vi "Claw Control.vi"() -> ()   [LabVIEW 2014]
doc: "This VI runs in parallel to other tasks. It can contain as many user-defined periodic loops as you need. These can carry out PID or other sorts of timed response."
uses:
  Vision/Robot Global Data.vi
  <vilib>/Rock Robotics/Network Tables/SD Write Number.vi
  <vilib>/Rock Robotics/Network Tables/SD Write Boolean.vi
panel:
  in  "PDB Channel":dbl
  out "Claw Motor Current Chart":dbl(graph)
  out "Time Request Running":u32
  out "Start Time":u32
  out "Prior Claw State":dbl
  out "Claw State":dbl=2.0
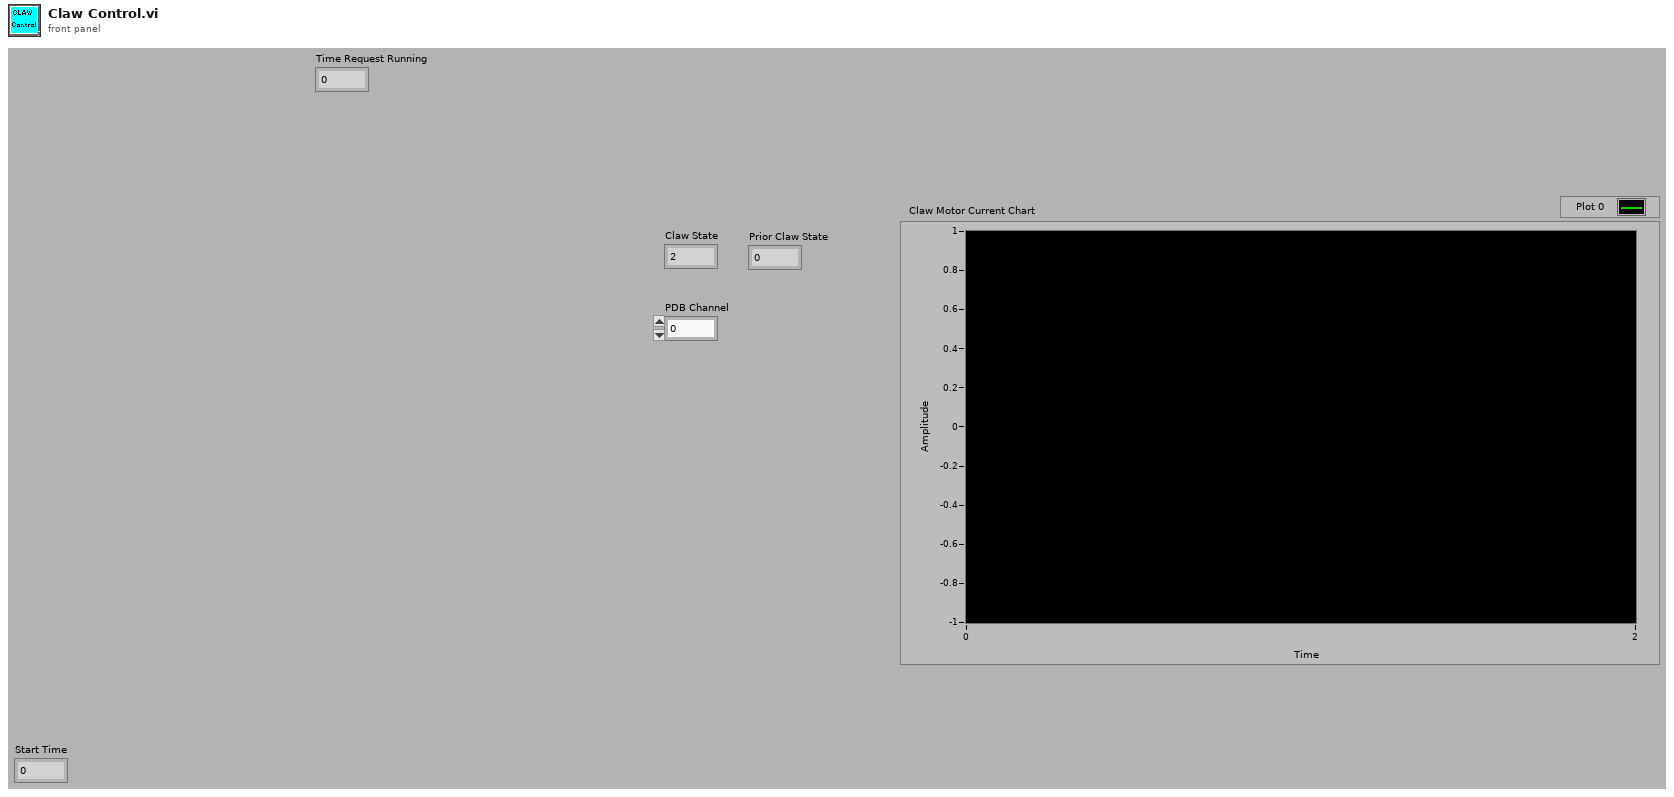
[diagram p1: front panel]
types:
  T1 = enum16{"Claw State Closing", "Claw State Closed"}
  T2 = enum16{"Claw State Opening", "Claw State Opened"}
  T3 = enum16{"Claw State Closing", "Claw State Closed", "Squeeze"}
  T4 = typedef "WPI_MotorControlDeviceRef.ctl" = cluster{"DeviceStatus":errorcluster, "Type":T5, "PWM":cluster{"Controller":T6, "PWM Channel":T7, "DeadBand":T8}, "CAN":cluster{"Device Number":u8, "Control Mode":T9, "Semaphore":T10, "Max Vout":dbl, "TalonSRX Control Mode":T11}, "Invert":bool, "TransformRef":T12, "InvTransformRef":T12}
  T5 = typedef "WPI_MotorControlType.ctl" = enum16{"PWM", "CAN", "CANTalonSRX"}
  T6 = typedef "FPGA_TypedefDigitalModule.ctl" = enum16{"Controller 1"}
  T7 = typedef "FPGA_DIOPWMChannel.ctl" = enum8{"PWM 0", "PWM 1", "PWM 2", "PWM 3", "PWM 4", "PWM 5", "PWM 6", "PWM 7", "PWM 8", "PWM 9", "PWM MXP 0", "PWM MXP 1", "PWM MXP 2", "PWM MXP 3", "PWM MXP 4", "PWM MXP 5", "PWM MXP 6", "PWM MXP 7", "PWM MXP 8", "PWM MXP 9", "Invalid"}
  T8 = typedef "WPI_PWMDeadband.ctl" = cluster{"Name":string, "maxPositivePwm":i32, "minPositivePwm":i32, "centerPwm":i32, "maxNegativePwm":i32, "minNegativePwm":i32, "angularRange":u16}
  T9 = typedef "WPI_CANJaguar_ControlMode.ctl" = enum8{"Percent VBus", "Current", "Speed", "Position", "Voltage"}
  T10 = typedef "Semaphore RefNum" = refnum<k1>
  T11 = typedef "WPI_CANTalonSRX_APIControlMode.ctl" = enum8{"Percent VBus", "Speed", "Position", "Slave", "Unchanged / Invalid"}
  T12 = typedef "WPI_PWMTransform_ConPane.ctl" = refnum<vi>
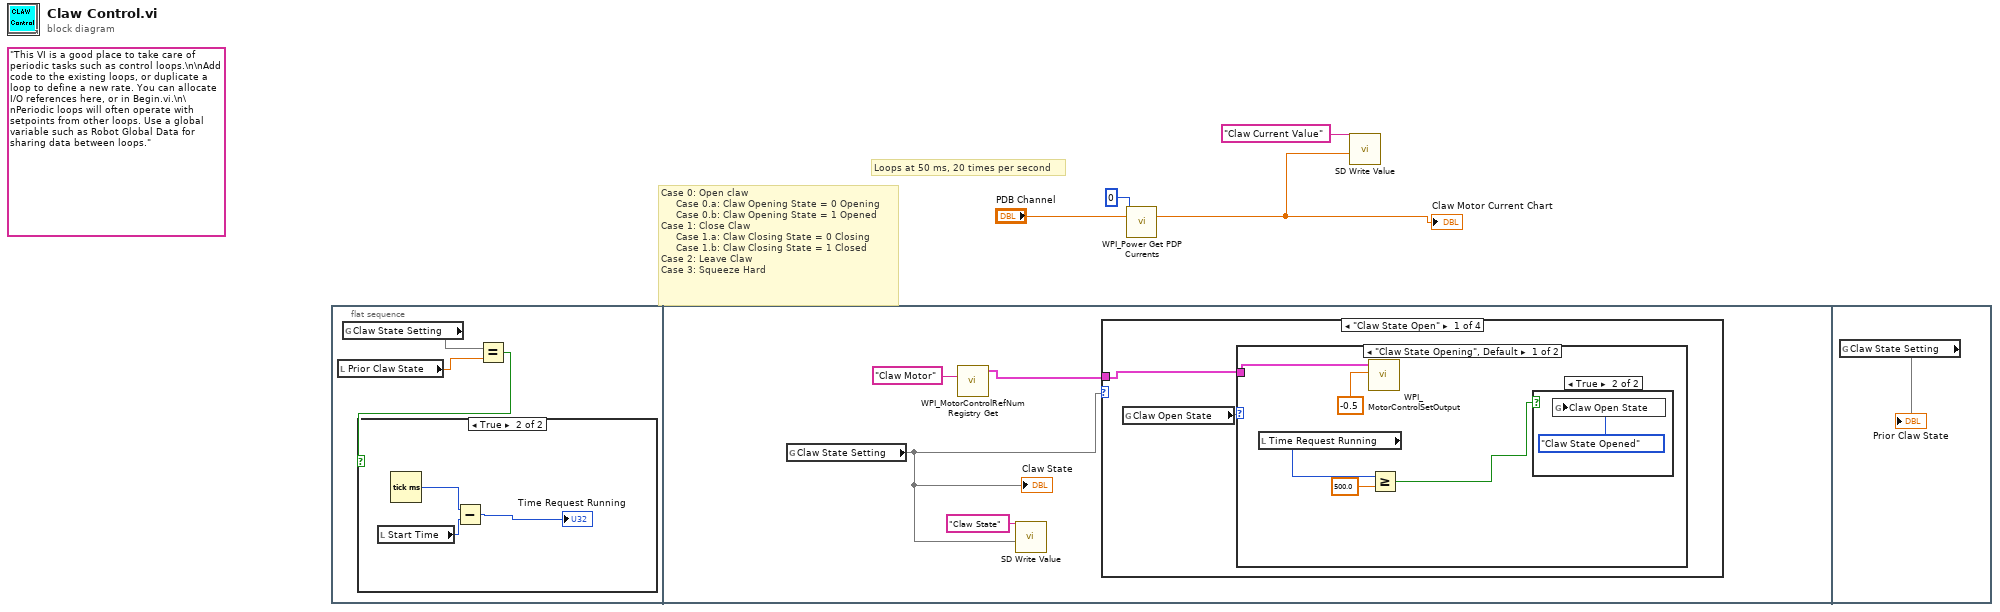
[diagram p0: block diagram]
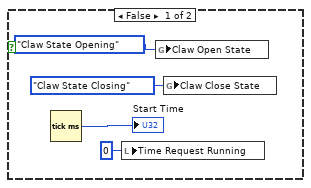
[diagram p2: hidden frame]
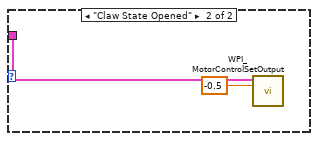
[diagram p4: hidden frame]
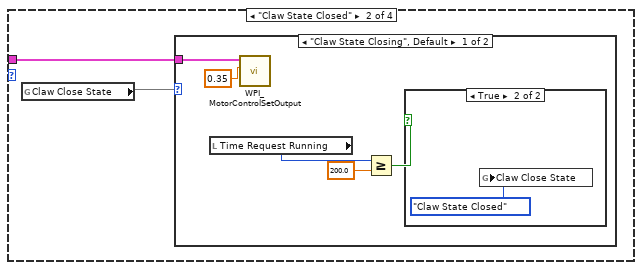
[diagram p5: hidden frame]
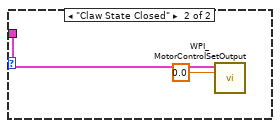
[diagram p7: hidden frame]
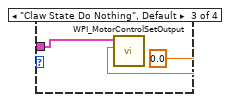
[diagram p8: hidden frame]
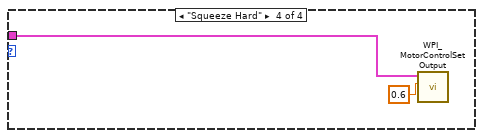
[diagram p9: hidden frame]
diagram:
  (unwired) "This VI is a good place to take care of periodic tasks such as control loops.\n\nAdd code to the existing loops, or duplicate a loop to define a new rate. You can allocate I/O references here, or in Begin.vi.\n\nPeriodic loops will often operate with setpoints from other loops. Use a global variable such as Robot Global Data for sharing data between loops."
  # "Case 0: Open claw\n     Case 0.a: Claw Opening State = 0 Opening\n     Case 0.b: Claw Opening State = 1 Opened\nCase 1: Close Claw \n     Case 1.a: Claw Closing State = 0 Closing\n     Case 1.b: Claw Closing State = 1 Closed\nCase 2: Leave Claw\nCase 3: Squeeze Hard"
  # "Loops at 50 ms, 20 times per second"
  n1 = flat-sequence {
    frame #0 {
      n2 = local read "Prior Claw State"() -> (w6:dbl)
      n3 = global read "Robot Global Data.vi" "Claw State Setting"() -> (w7)
      n4 = Equal?(x=w7, y=w6) -> (x = y?=w5:bool)
      n5 = case shown="True" w5 {
        frame False {
          n6 = Tick Count (ms)() -> (millisecond timer value=→"Start Time":u32)
          n7 = local write "Time Request Running"(u32 0 ("Time Request Running")) -> ()
          n8 = global write "Robot Global Data.vi" "Claw Open State"(T2."Claw State Opening" ("Claw Open State")) -> ()
          n9 = global write "Robot Global Data.vi" "Claw Close State"(T1."Claw State Closing" ("Claw Close State")) -> ()
        }
        frame True {
          n10 = local read "Start Time"() -> (w12:u32)
          n11 = Tick Count (ms)() -> (millisecond timer value=w13:u32)
          n12 = Subtract(x=w13, y=w12) -> (x-y=→"Time Request Running":u32)
        }
      }
    }
    frame #1 {
      n13 = global read "Robot Global Data.vi" "Claw State Setting"() -> (w15)
      "Claw State" <- w15
      n14 = call <vilib>:"WPI_MotorControlRefNum Registry Get.vi"("refnum name"="Claw Motor") -> ("MotorControlDevRef"=w17:T4)  [unwired: 9 in, 1 out]
      n15 = call-poly <vilib>:"SD Write Value.vi"("Boolean"=w15, "Name"="Claw State") -> ()  [unwired: 8 in, 2 out]
      n16 = case shown="\"Claw State Open\"" w15 {
        tunnel: w17 -> [w19 w30 w40 w42]
        frame "Claw State Open" {
          n17 = global read "Robot Global Data.vi" "Claw Open State"() -> (w20)
          n18 = case shown="\"Claw State Opening\", Default" w20 {
            tunnel: w19 -> [w25 w27]
            frame "Claw State Opening", Default {
              n19 = local read "Time Request Running"() -> (w22:u32)
              n20 = call <vilib>:"WPI_MotorControlSetOutput.vi"("Output"=-0.5, "MotorControlDevRef"=w25) -> ()  [unwired: 7 in, 3 out]
              n21 = Greater Or Equal?(x=w22, y=500.0) -> (x >= y?=w21:bool)
              n22 = case shown="True" w21 {
                frame False {
                }
                frame True {
                  n23 = global write "Robot Global Data.vi" "Claw Open State"(T2."Claw State Opened" ("Claw State Opening")) -> ()
                }
              }
            }
            frame "Claw State Opened" {
              n24 = call <vilib>:"WPI_MotorControlSetOutput.vi"("Output"=-0.5, "MotorControlDevRef"=w27) -> ()  [unwired: 7 in, 3 out]
            }
          }
        }
        frame "Claw State Closed" {
          n25 = global read "Robot Global Data.vi" "Claw Close State"() -> (w29)
          n26 = case shown="\"Claw State Closing\", Default" w29 {
            tunnel: w30 -> [w34 w37]
            frame "Claw State Closing", Default {
              n27 = local read "Time Request Running"() -> (w33:u32)
              n28 = call <vilib>:"WPI_MotorControlSetOutput.vi"("Output"=0.35, "MotorControlDevRef"=w34) -> ()  [unwired: 7 in, 3 out]
              n29 = Greater Or Equal?(x=w33, y=200.0) -> (x >= y?=w31:bool)
              n30 = case shown="True" w31 {
                frame False {
                }
                frame True {
                  n31 = global write "Robot Global Data.vi" "Claw Close State"(T3."Claw State Closed" ("Claw Close State")) -> ()
                }
              }
            }
            frame "Claw State Closed" {
              n32 = call <vilib>:"WPI_MotorControlSetOutput.vi"("Output"=0.0, "MotorControlDevRef"=w37) -> ()  [unwired: 7 in, 3 out]
            }
          }
        }
        frame "Claw State Do Nothing", Default {
          n33 = call <vilib>:"WPI_MotorControlSetOutput.vi"("Output"=0.0, "MotorControlDevRef"=w40) -> ()  [unwired: 7 in, 3 out]
        }
        frame "Squeeze Hard" {
          n34 = call <vilib>:"WPI_MotorControlSetOutput.vi"("Output"=0.6, "MotorControlDevRef"=w42) -> ()  [unwired: 7 in, 3 out]
        }
      }
    }
    frame #2 {
      n35 = global read "Robot Global Data.vi" "Claw State Setting"() -> (→"Prior Claw State")
    }
  }
  n36 = call <vilib>:"WPI_Power Get PDP Currents.vi"("Power Distribution Panel (0)"=u8 0, "PDP Channel"="PDB Channel") -> ("current (A)"=w1:dbl)  [unwired: 11 in, 2 out]
  "Claw Motor Current Chart" <- w1
  n37 = call-poly <vilib>:"SD Write Value.vi"("Numeric"=w1, "Name"="Claw Current Value") -> ()  [unwired: 8 in, 2 out]
